vi "enum.vi"() -> ()   [LabVIEW 2014]
doc: "A demo of the use of enumerator."
panel:
  in  "Stop":bool
  out "Output":dbl
  in  "Function":T1(ring)
  in  "B":dbl
  in  "A":dbl
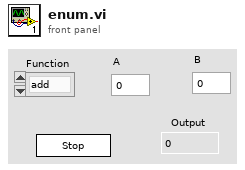
[diagram p1: front panel]
types:
  T1 = enum16{"add", "substract", "multiply", "divide", "square", "square root", "average", "max", "min"}
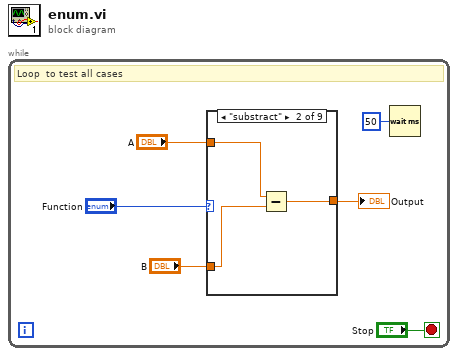
[diagram p0: block diagram]
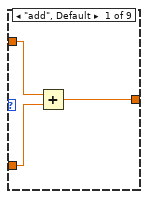
[diagram p2: hidden frame]
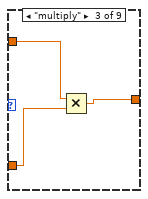
[diagram p3: hidden frame]
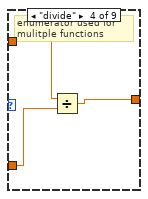
[diagram p4: hidden frame]
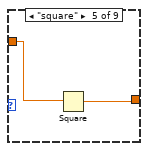
[diagram p5: hidden frame]
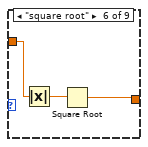
[diagram p6: hidden frame]
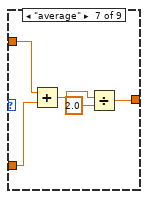
[diagram p7: hidden frame]
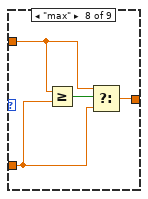
[diagram p8: hidden frame]
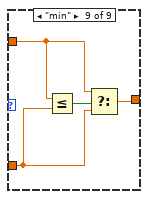
[diagram p9: hidden frame]
diagram:
  n1 = while {
    stop <- "Stop" stop-if-true
    # "Loop  to test all cases"
    n2 = case shown="\"substract\"" "Function" {
      tunnel: "A" -> [w9 w12 w15 w18 w20 w22 w26 w30 w34]
      tunnel: "B" -> [w8 w11 w14 w17 _ _ w25 w29 w33]
      tunnel: [w7 w10 w13 w16 w19 w23 w28 w32 w36] -> w1
      frame "add", Default {
        n3 = Add(x=w9, y=w8) -> (x+y=w7:dbl)
      }
      frame "substract" {
        n4 = Subtract(x=w12, y=w11) -> (x-y=w10:dbl)
      }
      frame "multiply" {
        n5 = Multiply(x=w15, y=w14) -> (x*y=w13:dbl)
      }
      frame "divide" {
        # "enumerator used for mulitple functions"
        n6 = Divide(x=w18, y=w17) -> (x/y=w16:dbl)
      }
      frame "square" {
        n7 = Square(x=w20) -> (x^2=w19:dbl)
      }
      frame "square root" {
        n8 = Absolute Value(x=w22) -> (abs(x)=w21:dbl)
        n9 = Square Root(x=w21) -> (sqrt(x)=w23:dbl)
      }
      frame "average" {
        n10 = Add(x=w26, y=w25) -> (x+y=w24:dbl)
        n11 = Divide(x=w24, y=2.0) -> (x/y=w28:dbl)
      }
      frame "max" {
        n12 = Greater Or Equal?(x=w30, y=w29) -> (x >= y?=w31:bool)
        n13 = Select(t=w30, s=w31, f=w29) -> (s? t:f=w32:dbl)
      }
      frame "min" {
        n14 = Less Or Equal?(x=w34, y=w33) -> (x <= y?=w35:bool)
        n15 = Select(t=w34, s=w35, f=w33) -> (s? t:f=w36:dbl)
      }
    }
    "Output" <- w1
    n16 = Wait (ms)(milliseconds to wait=u32 50) -> ()  [unwired: 1 out]
  }
